vi "Serialise Test.vi"() -> ()   [LabVIEW 2015, in "ByRef Variant Repository.lvlib"]
uses:
  ByRef Variant Repository.lvlib
panel:
  out "data":cluster{string, cluster{string, dbl, bool}}
  out "Value":bool
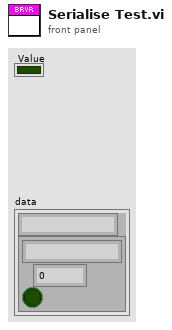
[diagram p1: front panel]
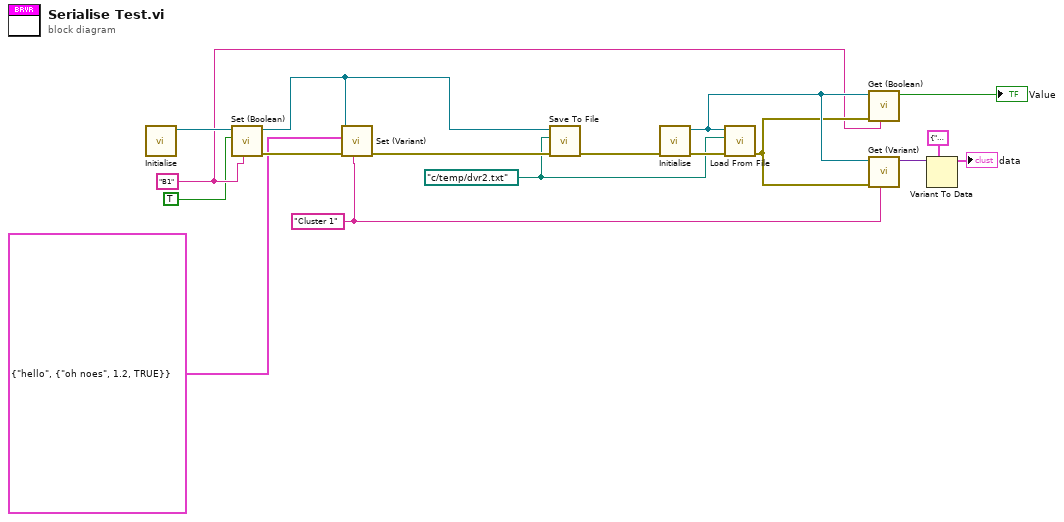
[diagram p0: block diagram]
diagram:
  w7 = path "c:/temp/dvr2.txt" ("File")
  w4 = "Cluster 1" ("Tag")
  w3 = "B1" ("Tag")
  n1 = call "Initialise.vi"() -> ("ByRef Variant Repsitory out"=w14:refnum<data-value>)  [unwired: 9 in, 1 out]
  n2 = call "Set (Boolean).vi"("Tag"=w3, "Value"=TRUE, "ByRef Variant Repsitory in"=w14) -> ("error out"=w15:errorcluster)  [unwired: 7 in]
  n3 = call "Set (Variant).vi"("Tag"=w4, "error in (no error)"=w15, "Value"=cluster{string, cluster{string, dbl, bool}} {"hello", {"oh noes", 1.2, TRUE}}, "ByRef Variant Repsitory in"=w14) -> ("error out"=w10:errorcluster)  [unwired: 6 in]
  n4 = call "Save To File.vi"("error in (no error)"=w10, "File"=w7, "ByRef Variant Repsitory in"=w14) -> ("error out"=w8:errorcluster)  [unwired: 7 in]
  n5 = call "Initialise.vi"("error in (no error)"=w8) -> ("error out"=w9:errorcluster, "ByRef Variant Repsitory out"=w6:refnum<data-value>)  [unwired: 8 in]
  n6 = call "Load From File.vi"("error in (no error)"=w9, "File"=w7, "ByRef Variant Repsitory in"=w6) -> ("error out"=w5:errorcluster)  [unwired: 7 in]
  n7 = call "Get (Boolean).vi"("Tag"=w3, "error in (no error)"=w5, "ByRef Variant Repsitory in"=w6) -> ("Value"=→"Value":bool)  [unwired: 6 in, 1 out]
  n8 = call "Get (Variant).vi"("Tag"=w4, "error in (no error)"=w5, "ByRef Variant Repsitory in"=w6) -> ("Value"=w13:variant)  [unwired: 6 in, 1 out]
  n9 = Variant To Data(type=cluster{string, cluster{string, dbl, bool}} {"", {"", 0.0, FALSE}}, Variant=w13) -> (data=→"data":cluster{string, cluster{string, dbl, bool}})  [unwired: 1 in, 1 out]
